vi "uActor_Core.vi"(8 "error in (no error)":errorcluster, 11 "uObserver in":refnum<class "uObserver.lvclass">) -> (0 "error out":errorcluster, 3 "uObserver out":refnum<class "uObserver.lvclass">)   [LabVIEW 2021, in "uFramework_pack_uActor.lvlib" / "uObserver.lvclass"]
uses:
  uObserver.lvclass
  uObserver.lvclass/uObserver.ctl
  Bin/uFramework.lvlibp/uActor/uActor.lvclass
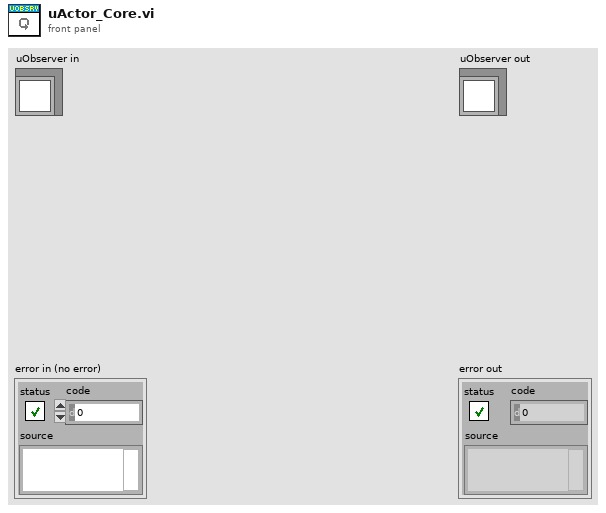
[diagram p1: front panel]
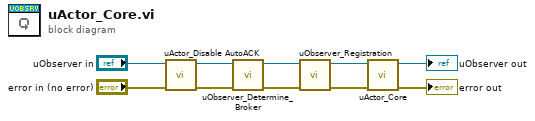
[diagram p0: block diagram]
diagram:
  n1 = call "uActor_Disable AutoACK.vi"("error in (no error)"="error in (no error)", "uActor in"="uObserver in") -> ("error out"=w3:errorcluster, "uActor out"=w1:refnum<class "uObserver.lvclass">)  [unwired: 8 in]
  n2 = call-dynamic "uObserver_Determine_Broker.vi"("error in (no error)"=w3, "uObserver in"=w1) -> ("error out"=w5:errorcluster, "uObserver out"=w4:refnum<class "uObserver.lvclass">)  [unwired: 8 in]
  n3 = call-dynamic "uObserver_Registration.vi"("error in (no error)"=w5, "uObserver in"=w4) -> ("error out"=w7:errorcluster, "uObserver out"=w6:refnum<class "uObserver.lvclass">)  [unwired: 8 in]
  n4 = call-parent "uActor_Core.vi"("error in (no error)"=w7, "uActor in"=w6) -> ("error out"=→"error out":errorcluster, "uActor out"=→"uObserver out":refnum<class "uObserver.lvclass">)  [unwired: 8 in]
